vi "SetItfClassCluster.vi"(8 "error in (no error)":errorcluster, 11 "Interface.lvclass":refnum<class "Interface.lvclass">) -> (0 "error out":errorcluster, 2 "Interface Class":T1={"Experiment.lvclass"=refnum, "DataFileName"=path "", "HdrFileName"=path "", "DataFileRef"=refnum, "ScanParams"={"Entête"="", "Scan list"=[], "NbCourbe"=1, "IndCourbe"=0, "NomDon"=["RTêta;", "X&Y;"], "Session "=0, "Date"="", "Time"="", "VarParams"=[], "UserName"="", "ScanTableSize"=[], "VarPar list"=[], "DescKeyword"=""}, "DataQRefs"=[], "XYGraphCurves"=[], "AllCurves"=[], "CurvesParams"=[], "ScanGphInd"=[], "CurvesSetup"=[], "ScanDataQ"=[], "GraphRefArr"=[], "Graph_FA"=[], "FirstFreeFA"=0, "GraphConfig"=0, "PanRef"=refnum, "FAGraphNumArr"=[], "BaseDataPath"=path "", "ListBoxRef"=refnum, "VarParCount"=0, "GraphQRefArr"=[], "XScalesNames"=[], "YScalesNames"=[], "MainGraphQ"=refnum, "GraphEvent"=refnum, "2DGraphQRefArr"=[], "Scan2DGphInd"=[], "2DGraphRefArr"=[], "2DGphParams"=[], "GraphNumbers"=[], "LastGrphNum"=0, "AllDataQ"=[], "AllQRefs"=[], "VarParQRefs"=[], "DatQIndex"=[], "CalcQIndex"=[], "SubVarParQRefs"=[], "AllVarParQ"=[], "UseSubFolder"=FALSE}, 3 "Interface.lvclass Out":refnum<class "Interface.lvclass">)   [LabVIEW 2019, in "Interface.lvclass"]
uses:
  Interface.lvclass
  ItfDataCluster.ctl
  Experiment Class/Experiment.lvclass
  ScanParams.ctl
  CurveSetup.ctl
  2DGraphSetup.ctl
  Interface.lvclass/Interface.ctl
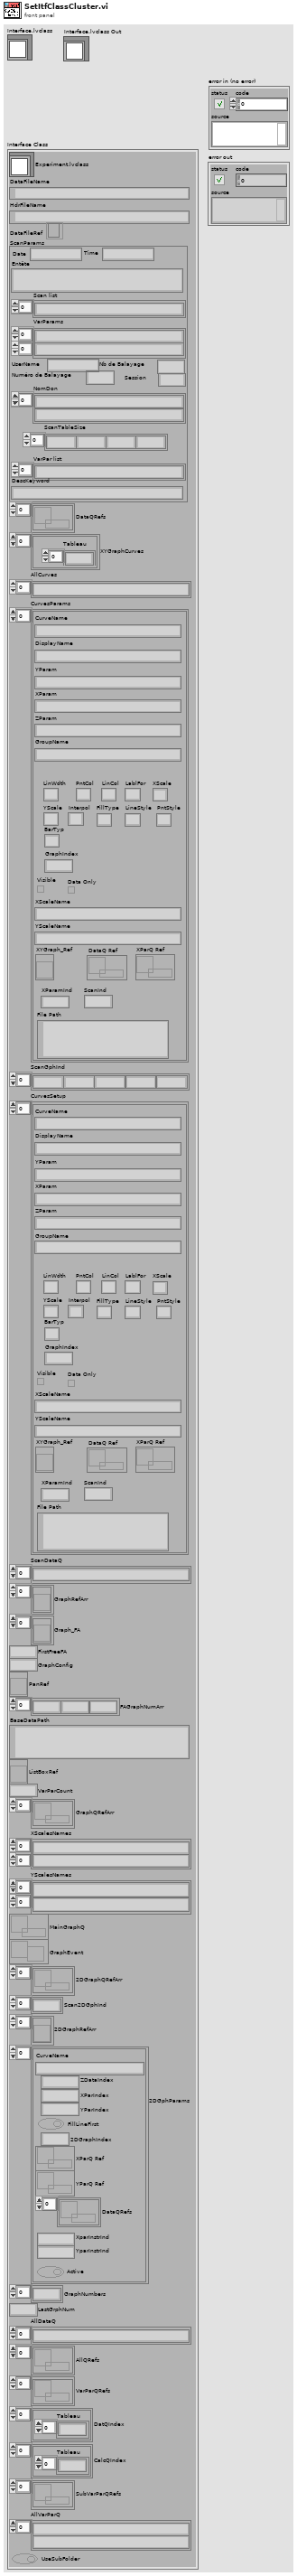
[diagram p1: front panel]
types:
  T1 = typedef "ItfDataCluster.ctl" = cluster{"Experiment.lvclass":refnum<class "Experiment.lvclass">, "DataFileName":path, "HdrFileName":path, "DataFileRef":refnum<file>, "ScanParams":T2, "DataQRefs":refnum<queue>[], "XYGraphCurves":cluster{"Tableau":i32[]}[], "AllCurves":string[], "CurvesParams":T3[], "ScanGphInd":i32[], "CurvesSetup":T3[], "ScanDataQ":string[], "GraphRefArr":refnum<vi>[], "Graph_FA":refnum<vi>[], "FirstFreeFA":u8, "GraphConfig":i32, "PanRef":refnum<vi>, "FAGraphNumArr":i32[], "BaseDataPath":path, "ListBoxRef":refnum<vi>, "VarParCount":i32, "GraphQRefArr":refnum<queue>[], "XScalesNames":string[][], "YScalesNames":string[][], "MainGraphQ":refnum<queue>, "GraphEvent":refnum<user-event>, "2DGraphQRefArr":refnum<queue>[], "Scan2DGphInd":i32[], "2DGraphRefArr":refnum<vi>[], "2DGphParams":T4[], "GraphNumbers":i32[], "LastGrphNum":i32, "AllDataQ":string[], "AllQRefs":refnum<queue>[], "VarParQRefs":refnum<queue>[], "DatQIndex":cluster{"Tableau":i32[]}[], "CalcQIndex":cluster{"Tableau":i32[]}[], "SubVarParQRefs":refnum<queue>[], "AllVarParQ":string[], "UseSubFolder":bool}
  T2 = typedef "Interface.lvclass/ScanParams.ctl" = cluster{"Entête":string, "Scan list":string[], "NbCourbe":i32, "IndCourbe":i64, "NomDon":string[], "Session ":i32, "Date":string, "Time":string, "VarParams":string[][], "UserName":string, "ScanTableSize":i32[], "VarPar list":string[], "DescKeyword":string}
  T3 = typedef "Interface.lvclass/CurveSetup.ctl" = cluster{"CurveName":string, "YParam":string, "XParam":string, "ZParam ":string, "GroupName":string, "LinWdth":u8, "PntCol":u32, "LinCol":u32, "LablFor":u8, "XScale":u32, "YScale":u32, "Interpol":u8, "DisplayName":string, "FillType":i16, "LineStyle":u8, "PntStyle":u8, "BarTyp":u8, "GraphIndex":i32, "Visible":bool, "XScaleName":string, "YScaleName":string, "XYGraph_Ref":refnum<vi>, "Data Only":bool, "DataQ Ref":refnum<queue>, "XParQ Ref":refnum<queue>, "XParamInd":i32, "ScanInd":i32, "File Path":path}
  T4 = typedef "2DGraphSetup.ctl" = cluster{"ZDataIndex":i32, "XParIndex":i32, "YParIndex":i32, "FillLineFirst":bool, "2DGraphIndex":i32, "XParQ Ref":refnum<queue>, "YParQ Ref":refnum<queue>, "DataQRefs":refnum<queue>[], "CurveName":string, "XparInstrInd":i32, "YparInstrInd":i32, "Active":bool}
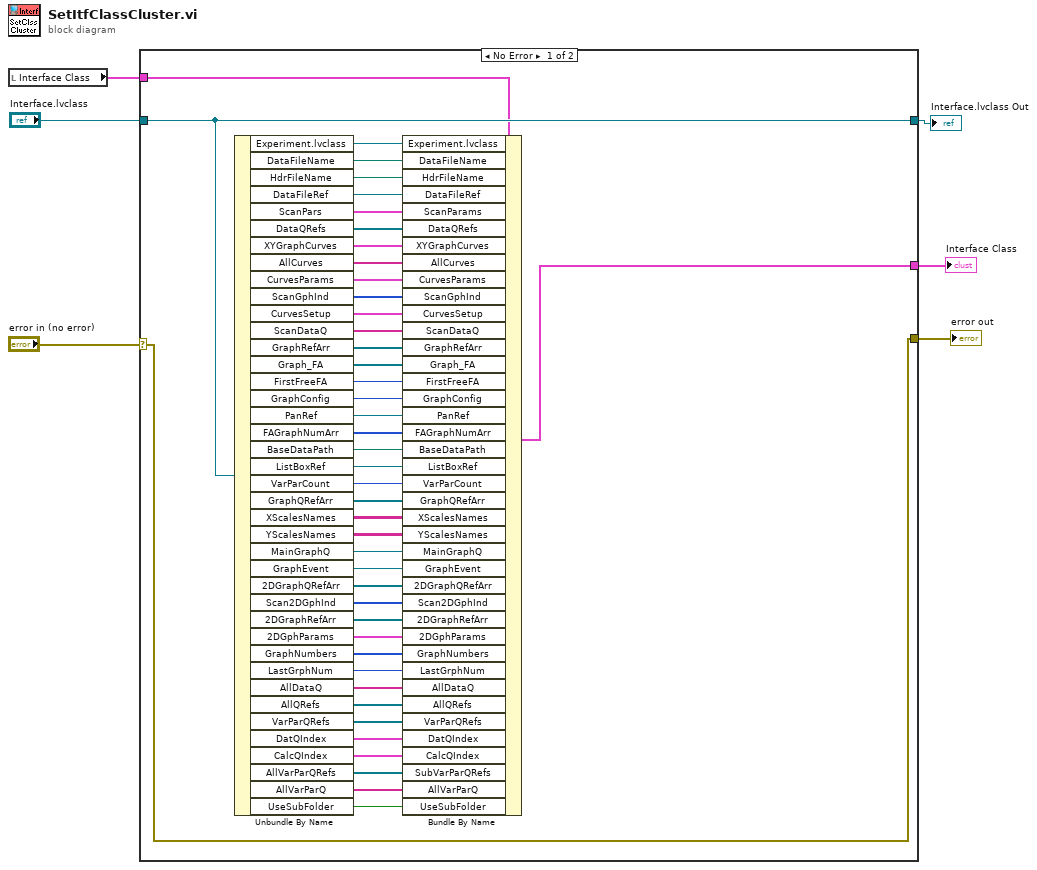
[diagram p0: block diagram]
diagram:
  n1 = local read "Interface Class"() -> (w2:T1)
  n2 = case shown="No Error" "error in (no error)" {
    selector: "error in (no error)" -> [w13 w53]
    tunnel: [w13 w53] -> w5
    tunnel: [w50 w52] -> w4
    tunnel: "Interface.lvclass" -> [w50 w52]
    tunnel: w2 -> [w49 w51]
    tunnel: [w14 w51] -> w1
    frame No Error {
      n3 = Unbundle By Name(w50) -> ("Experiment.lvclass"=w48:refnum<class "Experiment.lvclass">, "DataFileName"=w47:path, "HdrFileName"=w46:path, "DataFileRef"=w45:refnum<file>, "ScanPars"=w44:T2, "DataQRefs"=w43:refnum<queue>[], "XYGraphCurves"=w42:cluster{"Tableau":i32[]}[], "AllCurves"=w41:string[], "CurvesParams"=w40:T3[], "ScanGphInd"=w39:i32[], "CurvesSetup"=w38:T3[], "ScanDataQ"=w37:string[], "GraphRefArr"=w36:refnum<vi>[], "Graph_FA"=w35:refnum<vi>[], "FirstFreeFA"=w34:u8, "GraphConfig"=w33:i32, "PanRef"=w32:refnum<vi>, "FAGraphNumArr"=w31:i32[], "BaseDataPath"=w30:path, "ListBoxRef"=w29:refnum<vi>, "VarParCount"=w28:i32, "GraphQRefArr"=w27:refnum<queue>[], "XScalesNames"=w26:string[][], "YScalesNames"=w25:string[][], "MainGraphQ"=w24:refnum<queue>, "GraphEvent"=w23:refnum<user-event>, "2DGraphQRefArr"=w22:refnum<queue>[], "Scan2DGphInd"=w21:i32[], "2DGraphRefArr"=w20:refnum<vi>[], "2DGphParams"=w19:T4[], "GraphNumbers"=w18:i32[], "LastGrphNum"=w17:i32, "AllDataQ"=w16:string[], "AllQRefs"=w15:refnum<queue>[], "VarParQRefs"=w12:refnum<queue>[], "DatQIndex"=w11:cluster{"Tableau":i32[]}[], "CalcQIndex"=w10:cluster{"Tableau":i32[]}[], "AllVarParQRefs"=w8:refnum<queue>[], "AllVarParQ"=w9:string[], "UseSubFolder"=w7:bool)
      n4 = Bundle By Name(cluster=w49, "Experiment.lvclass"=w48, "DataFileName"=w47, "HdrFileName"=w46, "DataFileRef"=w45, "ScanParams"=w44, "DataQRefs"=w43, "XYGraphCurves"=w42, "AllCurves"=w41, "CurvesParams"=w40, "ScanGphInd"=w39, "CurvesSetup"=w38, "ScanDataQ"=w37, "GraphRefArr"=w36, "Graph_FA"=w35, "FirstFreeFA"=w34, "GraphConfig"=w33, "PanRef"=w32, "FAGraphNumArr"=w31, "BaseDataPath"=w30, "ListBoxRef"=w29, "VarParCount"=w28, "GraphQRefArr"=w27, "XScalesNames"=w26, "YScalesNames"=w25, "MainGraphQ"=w24, "GraphEvent"=w23, "2DGraphQRefArr"=w22, "Scan2DGphInd"=w21, "2DGraphRefArr"=w20, "2DGphParams"=w19, "GraphNumbers"=w18, "LastGrphNum"=w17, "AllDataQ"=w16, "AllQRefs"=w15, "VarParQRefs"=w12, "DatQIndex"=w11, "CalcQIndex"=w10, "SubVarParQRefs"=w8, "AllVarParQ"=w9, "UseSubFolder"=w7) -> (w14:T1)
    }
    frame Error {
    }
  }
  "error out" <- w5
  "Interface Class" <- w1
  "Interface.lvclass Out" <- w4
